vi "Acquire2_QPD3.6.vi"(1 "Save Data?":bool=TRUE, 2 "Calibrating?":bool, 5 "Main refnum":refnum<file>, 7 "error in":errorcluster, 11 "Trap ref":refnum<file>, 13 "data array":dbl[][](array[numeric])) -> (20 "all data 2":dbl[][](array[numeric]), 21 "QPD data":dbl[][](array[numeric]), 24 "dup refnum":refnum<file>, 27 "error out":errorcluster)   [LabVIEW 2016]
uses:
  <vilib>/Analysis/baseanly.llb/Mean (DBL).vi
  <vilib>/Analysis/NI_AALBase.lvlib
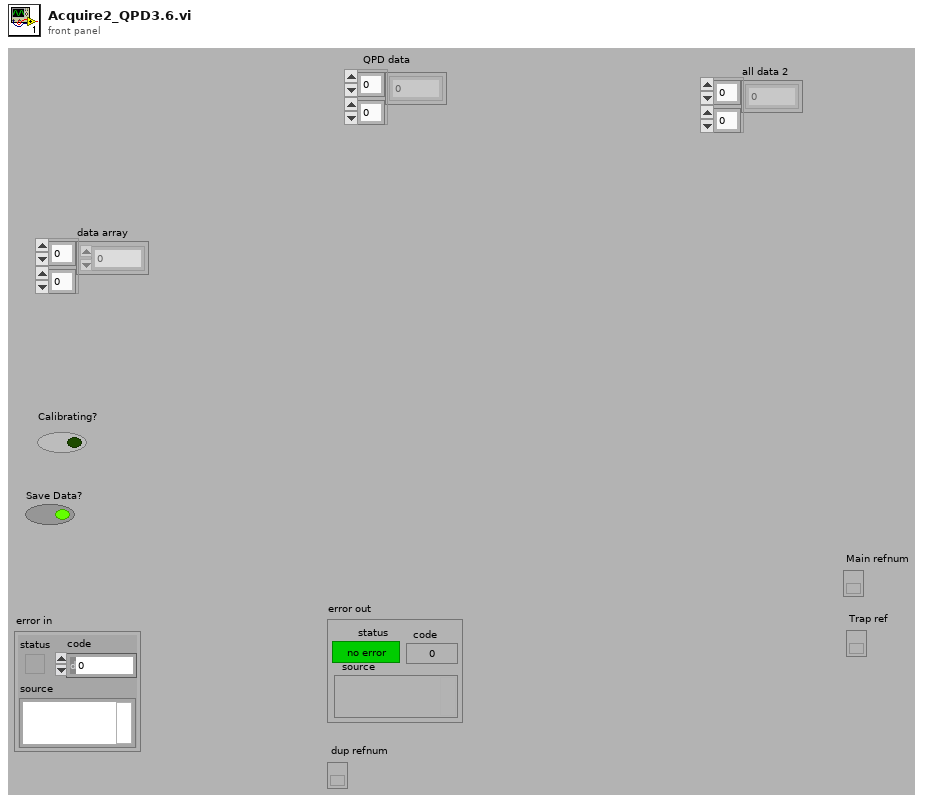
[diagram p1: front panel]
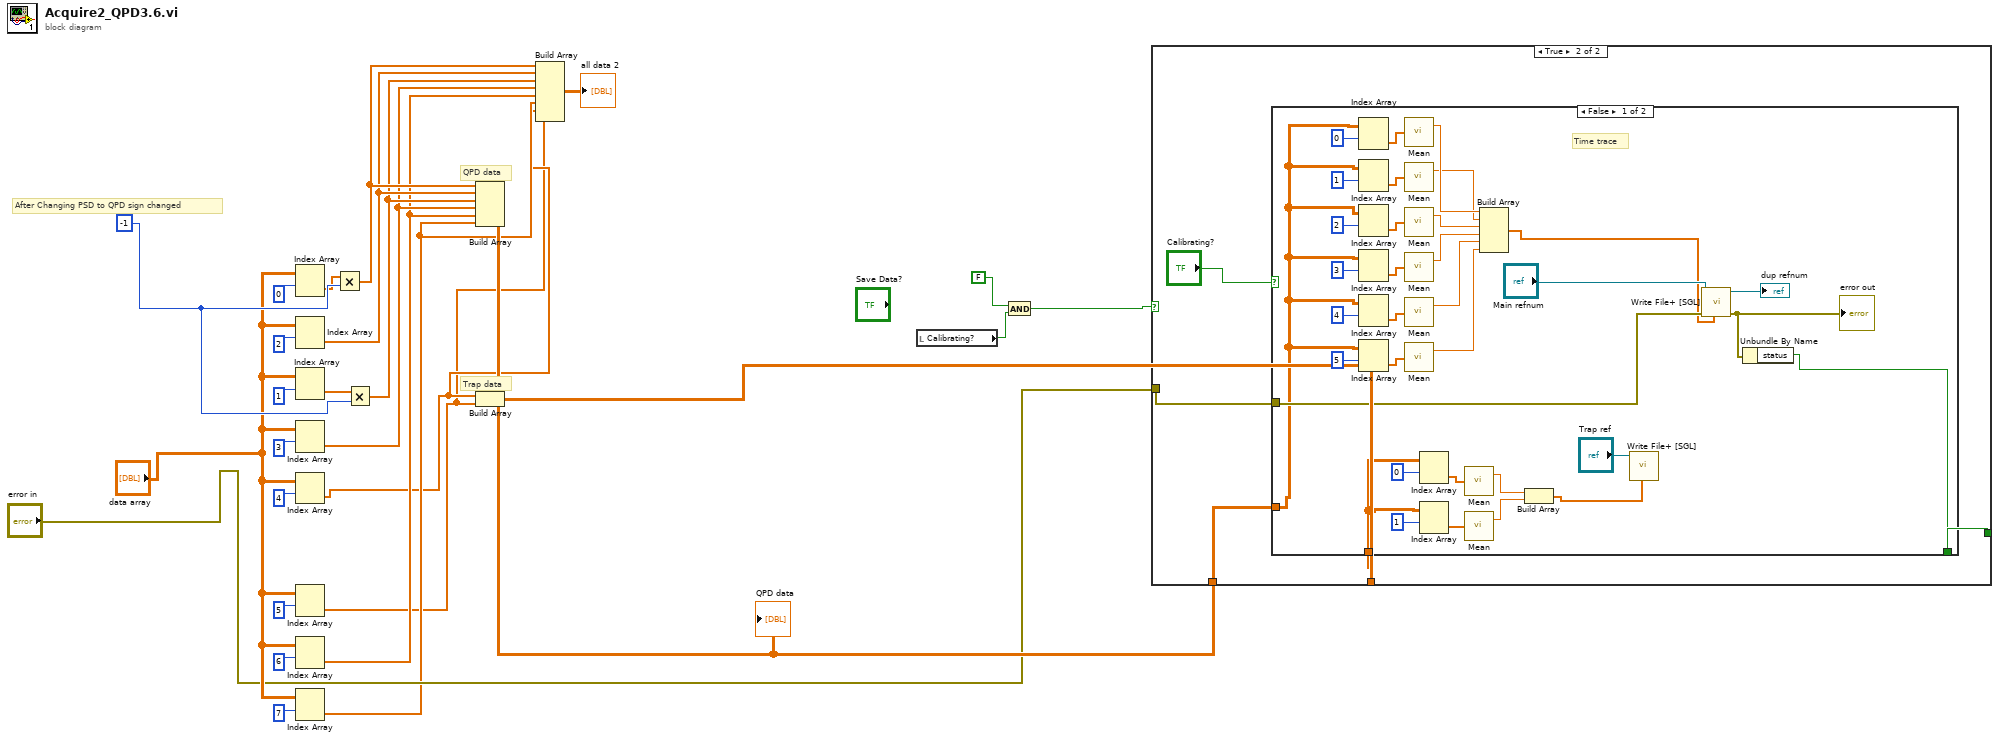
[diagram p0: block diagram]
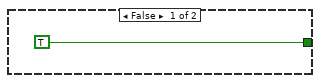
[diagram p2: hidden frame]
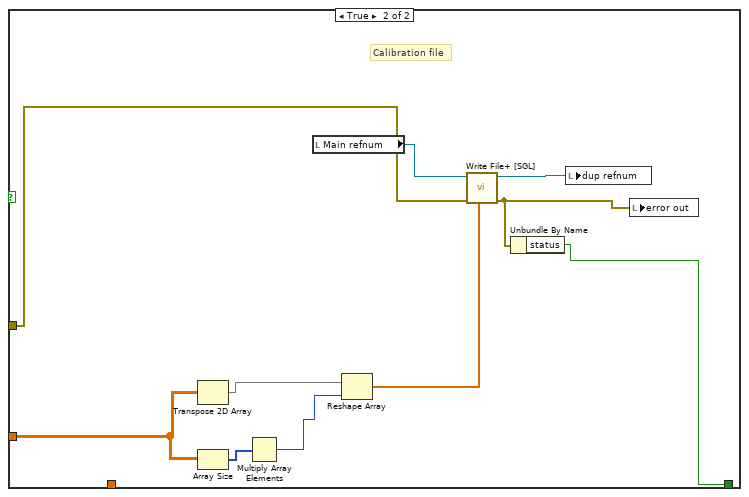
[diagram p3: hidden frame]
diagram:
  w19 = -1
  # "Trap data"
  # "QPD data"
  # "After Changing PSD to QPD sign changed"
  n1 = Index Array(array="data array", index (row)=0 ("disabled index (col)")) -> (element=w18:dbl[])  [unwired: 1 in]
  n2 = Index Array(array="data array", index (row)=2 ("disabled index (col)")) -> (element=w9:dbl[])  [unwired: 1 in]
  n3 = Index Array(array="data array", index (row)=1 ("disabled index (col)")) -> (element=w15:dbl[])  [unwired: 1 in]
  n4 = Index Array(array="data array", index (row)=3 ("disabled index (col)")) -> (element=w7:dbl[])  [unwired: 1 in]
  n5 = Index Array(array="data array", index (row)=4 ("disabled index (col)")) -> (element=w4:dbl[])  [unwired: 1 in]
  n6 = Index Array(array="data array", index (row)=5 ("disabled index (col)")) -> (element=w3:dbl[])  [unwired: 1 in]
  n7 = Index Array(array="data array", index (row)=6 ("disabled index (col)")) -> (element=w6:dbl[])  [unwired: 1 in]
  n8 = Index Array(array="data array", index (row)=7 ("disabled index (col)")) -> (element=w5:dbl[])  [unwired: 1 in]
  n9 = Multiply(x=w18, y=w19) -> (x*y=w10:dbl[])
  n10 = Multiply(x=w15, y=w19) -> (x*y=w8:dbl[])
  n11 = Build Array(w10, w9, w8, w7, w6, w5) -> (w14:dbl[][])
  "QPD data" <- w14
  n12 = Build Array(w4, w3) -> (w13:dbl[][])
  n13 = Build Array(w10, w9, w8, w7, w6, w5, w4, w3) -> (→"all data 2":dbl[][])
  n14 = local read "Calibrating?"() -> (w16:bool)
  n15 = And(x=FALSE, y=w16) -> (x .and. y?=w17:bool)
  n16 = case shown="True" w17 {
    tunnel: [TRUE ("status") w33] -> _
    tunnel: "error in" -> [_ w32]
    tunnel: w14 -> [_ w31]
    tunnel: w13 -> [_ w29]
    frame False {
    }
    frame True {
      n17 = case shown="False" "Calibrating?" {
        tunnel: [w67 w77] -> w33
        tunnel: w32 -> [w65 w76]
        tunnel: w31 -> [w46 w71]
        tunnel: w29 -> [w34 _]
        frame False {
          # "Time trace"
          n18 = Index Array(array=w46, index (row)=0) -> (element=w56:dbl[])  [unwired: 1 in]
          n19 = Index Array(array=w46, index (row)=1) -> (element=w55:dbl[])  [unwired: 1 in]
          n20 = Index Array(array=w46, index (row)=2) -> (element=w54:dbl[])  [unwired: 1 in]
          n21 = Index Array(array=w46, index (row)=3) -> (element=w53:dbl[])  [unwired: 1 in]
          n22 = Index Array(array=w46, index (row)=4) -> (element=w52:dbl[])  [unwired: 1 in]
          n23 = Index Array(array=w46, index (row)=5) -> (element=w51:dbl[])  [unwired: 1 in]
          n24 = call-poly <vilib>:"Mean.vi"("X"=w56) -> ("mean"=w50:dbl)  [unwired: 1 out]
          n25 = call-poly <vilib>:"Mean.vi"("X"=w55) -> ("mean"=w45:dbl)  [unwired: 1 out]
          n26 = call-poly <vilib>:"Mean.vi"("X"=w54) -> ("mean"=w49:dbl)  [unwired: 1 out]
          n27 = call-poly <vilib>:"Mean.vi"("X"=w53) -> ("mean"=w48:dbl)  [unwired: 1 out]
          n28 = call-poly <vilib>:"Mean.vi"("X"=w52) -> ("mean"=w47:dbl)  [unwired: 1 out]
          n29 = call-poly <vilib>:"Mean.vi"("X"=w51) -> ("mean"=w44:dbl)  [unwired: 1 out]
          n30 = Index Array(array=w34, index (row)=0) -> (element=w38:dbl[])  [unwired: 1 in]
          n31 = Index Array(array=w34, index (row)=1) -> (element=w39:dbl[])  [unwired: 1 in]
          n32 = call-poly <vilib>:"Mean.vi"("X"=w38) -> ("mean"=w40:dbl)  [unwired: 1 out]
          n33 = call-poly <vilib>:"Mean.vi"("X"=w39) -> ("mean"=w41:dbl)  [unwired: 1 out]
          n34 = Build Array(w50, w45, w49, w48, w47, w44) -> (w43:dbl[])
          n35 = Build Array(w40, w41) -> (w42:dbl[])
          n36 = call <vilib>:"Write File+ [SGL].vi"("1D array"=w42, "refnum"="Trap ref") -> ()  [unwired: 7 in, 3 out]
          n37 = call <vilib>:"Write File+ [SGL].vi"("1D array"=w43, "error in (no error)"=w65, "refnum"="Main refnum") -> ("error out"=w66:errorcluster, "dup refnum"=→"dup refnum":refnum<file>)  [unwired: 6 in, 1 out]
          "error out" <- w66
          n38 = Unbundle By Name(w66) -> ("status"=w67:bool)
        }
        frame True {
          # "Calibration file"
          n39 = Transpose 2D Array(2D array=w71) -> (transposed array=w73:dbl[][])
          n40 = Array Size(array=w71) -> (size(s)=w74:i32[])
          n41 = Multiply Array Elements(1:w74) -> (0:w72:i32)
          n42 = local read "Main refnum"() -> (w75:refnum<file>)
          n43 = Reshape Array(w73, w72) -> (w70:dbl[])
          n44 = call <vilib>:"Write File+ [SGL].vi"("1D array"=w70, "error in (no error)"=w76, "refnum"=w75) -> ("error out"=w68:errorcluster, "dup refnum"=w69:refnum<file>)  [unwired: 6 in, 1 out]
          n45 = Unbundle By Name(w68) -> ("status"=w77:bool)
          n46 = local write "dup refnum"(w69) -> ()
          n47 = local write "error out"(w68) -> ()
        }
      }
    }
  }
